vi "PID setting LHS RHS FGV.vi"(7 "Command":T2(ring), 8 "error in (no error)":errorcluster, 9 "PID gains":T1, 11 "File Path":path) -> (0 "error out":errorcluster, 2 "PID gains":T1)   [LabVIEW 2018]
doc: "This Subvi usde for CSV Initialize ,Read, Write and close.\nIntilise case; we check File avaliblity in not found create csv file\nRead Case ; Read data from csv file"
uses:
  <vilib>/Utility/file.llb/Write Delimited Spreadsheet (string).vi
  <vilib>/Utility/file.llb/Read Delimited Spreadsheet (string).vi
panel:
  # "LHS\nRHS"
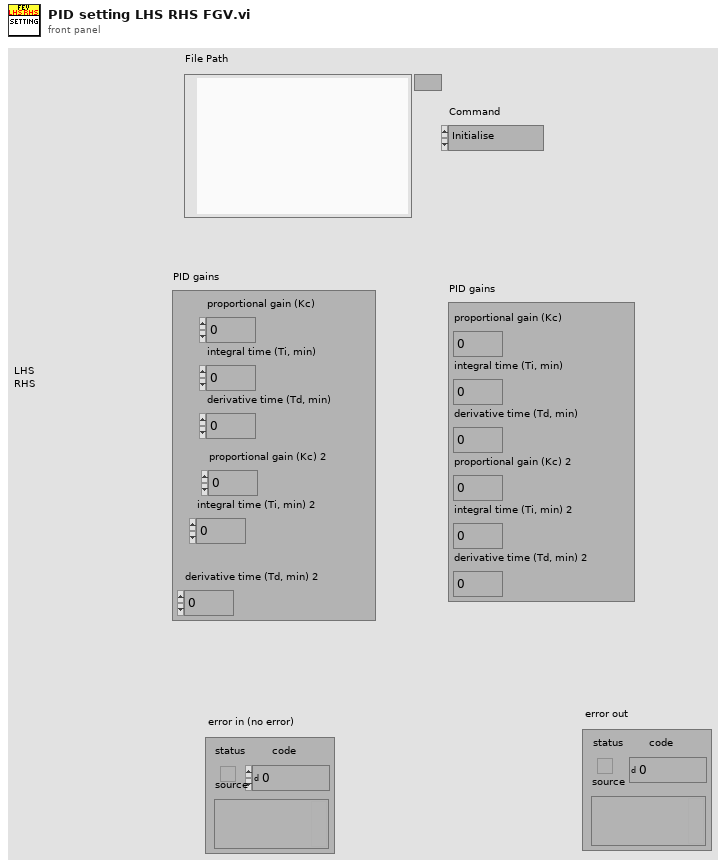
[diagram p1: front panel]
types:
  T1 = cluster{"proportional gain (Kc)":dbl, "integral time (Ti, min)":dbl, "derivative time (Td, min)":dbl, "proportional gain (Kc) 2":dbl, "integral time (Ti, min) 2":dbl, "derivative time (Td, min) 2":dbl}
  T2 = enum16{"Initialise", "Read Data", "Write Data", "Close"}
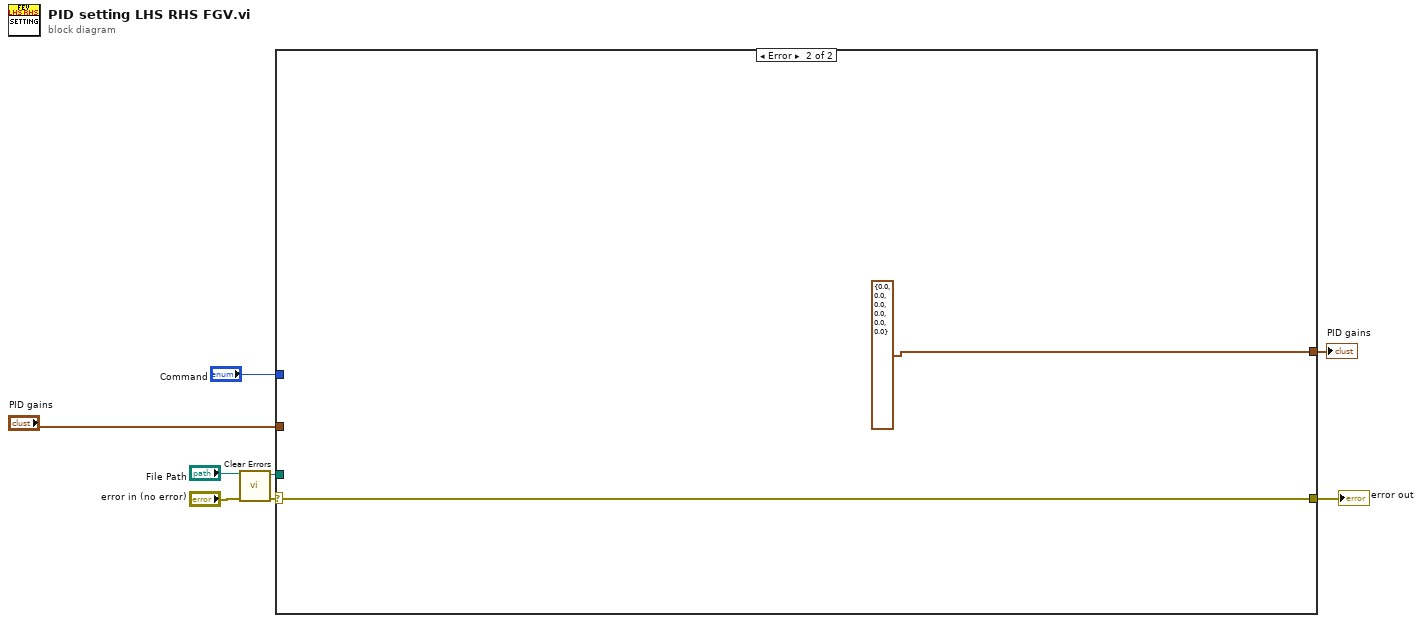
[diagram p0: block diagram]
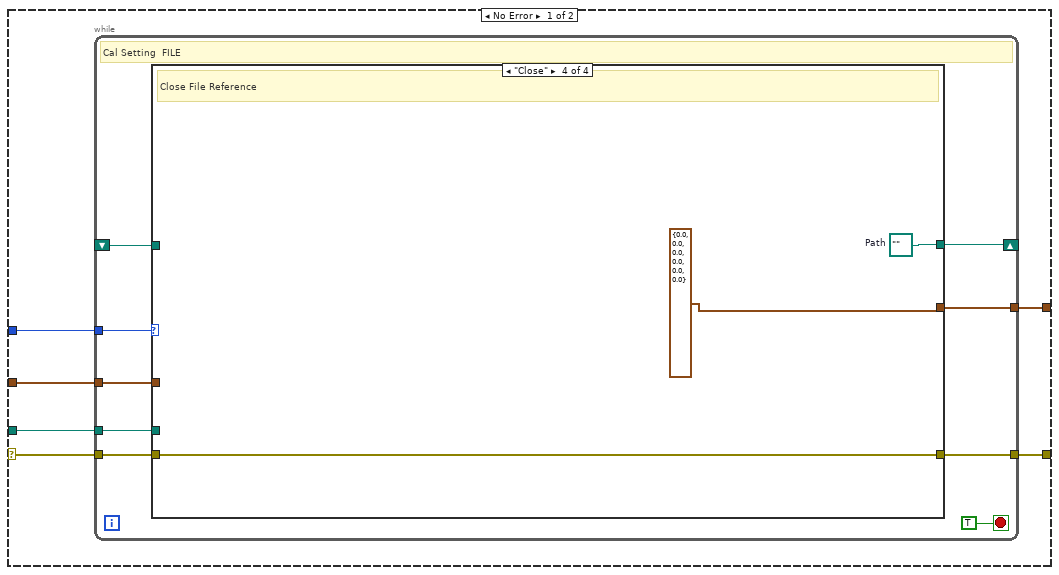
[diagram p2: hidden frame]
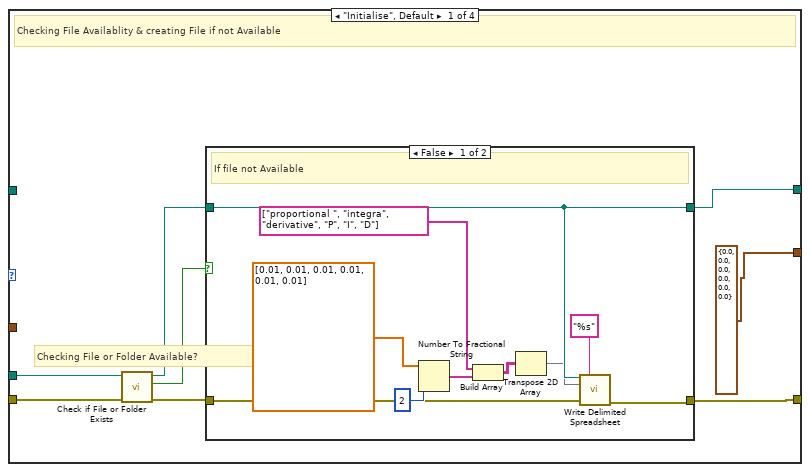
[diagram p3: hidden frame]
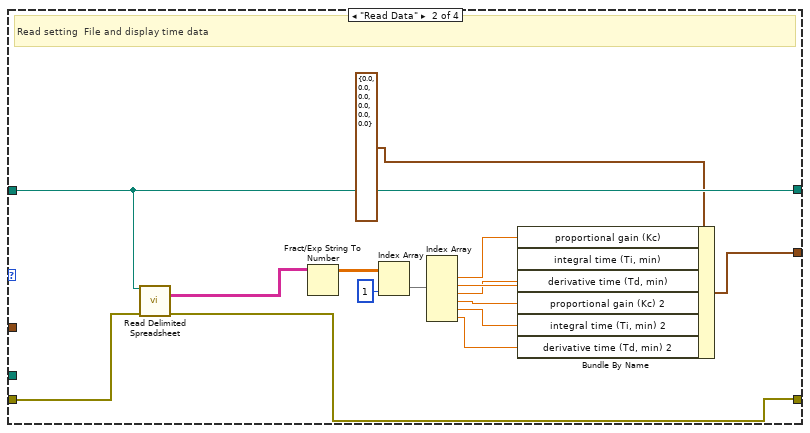
[diagram p5: hidden frame]
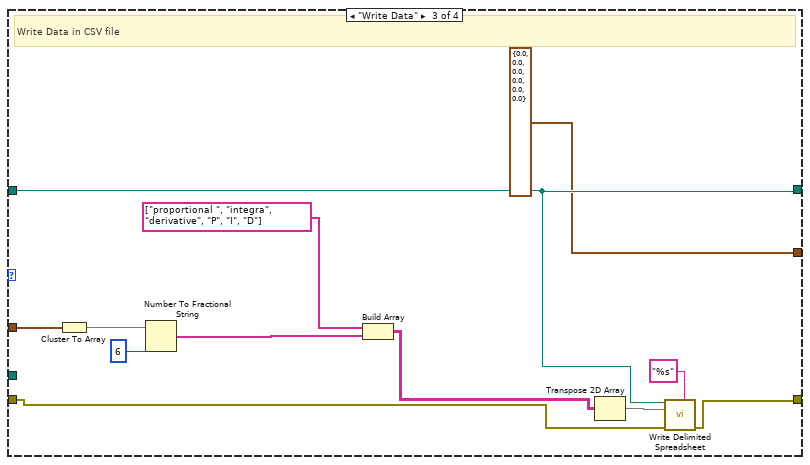
[diagram p6: hidden frame]
diagram:
  n1 = call <vilib>:"Clear Errors.vi"("error in (no error)"="error in (no error)") -> ("error out"=w3:errorcluster)  [unwired: 5 in, 1 out]
  n2 = case shown="Error" w3 {
    selector: w3 -> [w12 w74]
    tunnel: [w11 w74] -> w6
    tunnel: "Command" -> [w13 _]
    tunnel: "File Path" -> [w10 _]
    tunnel: "PID gains" -> [w9 _]
    tunnel: [w8 T1 {"proportional gain (Kc)"=0.0, "integral time (Ti, min)"=0.0, "derivative time (Td, min)"=0.0, "proportional gain (Kc) 2"=0.0, "integral time (Ti, min) 2"=0.0, "derivative time (Td, min) 2"=0.0} ("PID gains")] -> w1
    frame No Error {
      n3 = while {
        shift-right: [w17] -> _
        shift-left: _ -> [w16]
        tunnel: w13 -> [w21]
        tunnel: w12 -> [w20]
        tunnel: [w19] -> w11
        tunnel: w10 -> [w18]
        tunnel: w9 -> [w15]
        tunnel: [w14] -> w8
        stop <- TRUE stop-if-true
        # "Cal Setting  FILE"
        n4 = case shown="\"Close\"" w21 {
          tunnel: w20 -> [w30 w55 w62 w72]
          tunnel: [w24 w54 w61 w72] -> w19
          tunnel: w18 -> [w29 _ _ _]
          tunnel: [w27 w56 w60 w71] -> w17
          tunnel: w16 -> [_ w56 w60 _]
          tunnel: w15 -> [_ _ w69 _]
          tunnel: [T1 {"proportional gain (Kc)"=0.0, "integral time (Ti, min)"=0.0, "derivative time (Td, min)"=0.0, "proportional gain (Kc) 2"=0.0, "integral time (Ti, min) 2"=0.0, "derivative time (Td, min) 2"=0.0} ("PID gains") w44 T1 {"proportional gain (Kc)"=0.0, "integral time (Ti, min)"=0.0, "derivative time (Td, min)"=0.0, "proportional gain (Kc) 2"=0.0, "integral time (Ti, min) 2"=0.0, "derivative time (Td, min) 2"=0.0} ("PID gains") T1 {"proportional gain (Kc)"=0.0, "integral time (Ti, min)"=0.0, "derivative time (Td, min)"=0.0, "proportional gain (Kc) 2"=0.0, "integral time (Ti, min) 2"=0.0, "derivative time (Td, min) 2"=0.0} ("PID gains")] -> w14
          frame "Initialise", Default {
            # "Checking File or Folder Available?"
            # "Checking File Availablity & creating File if not Available"
            n5 = call <vilib>:"Check if File or Folder Exists.vi"("error in (no error)"=w30, "path"=w29) -> ("error out"=w25:errorcluster, "file or folder exists?"=w28:bool, "dup path"=w26:path)  [unwired: 7 in]
            n6 = case shown="False" w28 {
              tunnel: [w35 w42] -> w27
              tunnel: w26 -> [w35 w42]
              tunnel: w25 -> [w32 w41]
              tunnel: [w31 w41] -> w24
              frame False {
                # "If file not Available"
                n7 = Number To Fractional String(number=dbl[] [0.01, 0.01, 0.01, 0.01, 0.01, 0.01], precision (6)=i16 2) -> (F-format string=w39:string[])  [unwired: 2 in]
                n8 = Build Array(string[] ["proportional ", "integra", "derivative", "P", "I", "D"] ("element"), w39) -> (w40:string[][])
                n9 = Transpose 2D Array(2D array=w40) -> (transposed array=w34:string[][])
                n10 = call-poly <vilib>:"Write Delimited Spreadsheet.vi"("file path (dialog if empty)"=w35, "format (%s)"="%s", "2D data"=w34, "error in (no error)"=w32) -> ("error out"=w31:errorcluster)  [unwired: 10 in, 1 out]
              }
              frame True {
                # "If File available"
              }
            }
          }
          frame "Read Data" {
            # "Read setting  File and display time data"
            n11 = call-poly <vilib>:"Read Delimited Spreadsheet.vi"("file path (dialog if empty)"=w56, "error in (no error)"=w55) -> ("all rows"=w52:string[][], "error out"=w54:errorcluster)  [unwired: 8 in, 4 out]
            n12 = Fract/Exp String To Number(string=w52) -> (number=w51:dbl[][])  [unwired: 3 in, 1 out]
            n13 = Index Array(array=w51, index (col)=1 ("disabled index (col)")) -> (element=w53:dbl[])  [unwired: 1 in]
            n14 = Index Array(array=w53) -> (element #1=w50:dbl, element #2=w49:dbl, element #3=w48:dbl, element #4=w47:dbl, element #5=w46:dbl, element #6=w45:dbl)  [unwired: 6 in]
            n15 = Bundle By Name(cluster=T1 {"proportional gain (Kc)"=0.0, "integral time (Ti, min)"=0.0, "derivative time (Td, min)"=0.0, "proportional gain (Kc) 2"=0.0, "integral time (Ti, min) 2"=0.0, "derivative time (Td, min) 2"=0.0} ("PID gains"), "proportional gain (Kc)"=w50, "integral time (Ti, min)"=w49, "derivative time (Td, min)"=w48, "proportional gain (Kc) 2"=w47, "integral time (Ti, min) 2"=w46, "derivative time (Td, min) 2"=w45) -> (w44:T1)
          }
          frame "Write Data" {
            # "Write Data in CSV file"
            n16 = Cluster To Array(cluster=w69) -> (array=w65:dbl[])
            n17 = Number To Fractional String(number=w65, precision (6)=i16 6) -> (F-format string=w68:string[])  [unwired: 2 in]
            n18 = Build Array(string[] ["proportional ", "integra", "derivative", "P", "I", "D"] ("element"), w68) -> (w59:string[][])
            n19 = Transpose 2D Array(2D array=w59) -> (transposed array=w64:string[][])
            n20 = call-poly <vilib>:"Write Delimited Spreadsheet.vi"("file path (dialog if empty)"=w60, "format (%s)"="%s", "2D data"=w64, "error in (no error)"=w62) -> ("error out"=w61:errorcluster)  [unwired: 10 in, 1 out]
          }
          frame "Close" {
            w71 = path ""  # Path
            # "Close File Reference"
          }
        }
      }
    }
    frame Error {
    }
  }
  "error out" <- w6
  "PID gains" <- w1
